vi "GPS显示界面.vi"() -> ()   [LabVIEW 2016, in "环境动力监测库.lvlib" / "NMEA.lvlib"]
uses:
  NMEA.lvlib
  NMEA_GPVTG-data.ctl
  NMEA_Mode.ctl
  NMEA_GPRMC-data.ctl
  NMEA_LatitudeDirection.ctl
  NMEA_LongitudeDirection.ctl
  NMEA_GPGGA-data.ctl
  NMEA_GPS-Quality.ctl
  <vilib>/Utility/miscctls.llb/LVPointTypeDef.ctl
  <vilib>/Utility/config.llb/NI_LVConfig.lvlib
panel:
  in  "解除告警":bool
  out "x+1":u32
  out "浮标定位点":cluster{"纬度":dbl, "经度":dbl}
  out "Port":string
  out "IP":string
  in  "手动设置定位":bool caption="定位自动获取OFF/手动设置ON"
  out "波特率":u32
  out "串口":string
  in  "移位报警设定值":dbl=1000.0
  out "GPS-Quality":T1
  out "定位状态":bool=TRUE
  in  "配置":bool
  out "Coordinates":picture
  in  "reset odometer":bool
  out "方位角 (deg)":dbl(knob) scale=0.0..360.0
  out "偏移量/米":dbl format="%#.2f"
  out "水平运动速度 (km/h)":dbl(knob) scale=0.0..180.0
  out "海拔":dbl format="%.2f"
  out "纬度":dbl
  out "经度":dbl
  out "时间":timestamp format="%<%H:%M:%S>T"
  out "日期":timestamp format="%<%Y/%m/%d>T"
  out "$GPGGA-message_OUT":T2={"TimeStamp"=timestamp(0 s since 1904-01-01), "Latitude"=0.0, "Latitude-Direction"=enum."", "Longitude"=1.0, "Longitude-Direction"=enum."", "GPS-Quality"=enum."GPS fix (SPS)", "Number of Satellites"=0, "Horizontal Dilution of Precision"=0.0, "Altitude above Mean-Sea-Level"=0.0, "Geoidal separation"=0.0, "Time since last DGPS update"=0.0, "DGPS reference station ID"=0} {"Time since last DGPS update" format="%.02f [s]"; "Geoidal separation" format="%.02f [m]"; "Altitude above Mean-Sea-Level" format="%.02f [m]"; "Horizontal Dilution of Precision" format="%.02f [HDOP]"; "Longitude" format="%0.4f [long]"; "Latitude" format="%.04f [lat]"; "TimeStamp" format="%<%.2X>T"}
  out "$GPRMC-message_OUT":T5={"TimeStamp"=timestamp(0 s since 1904-01-01), "Validity"=FALSE, "Latitude"=0.0, "Latitude-Direction"=enum."North", "Longitude"=0.0, "Longitude-Direction"=enum."East", "Speed in knots"=0.0, "True course"=0.0, "Date Stamp"=timestamp(0 s since 1904-01-01), "Magnetic Variation (East/West)"=0.0} {"Magnetic Variation (East/West)" format="%.02f [deg]"; "Date Stamp" format="%<%x>T"; "True course" format="%.02f [deg]"; "Speed in knots" format="%.02f [kts]"; "Longitude" format="%0.4f [long]"; "Latitude" format="%.04f [lat]"; "TimeStamp" format="%<%.2X>T"}
  out "$GPVTG-message_OUT":T6={"True Course over Ground"=0.0, "Magnetic Course over Ground"=0.0, "Speed over Ground in knots"=0.0, "Speed over Ground in km/h"=1.0, "Mode"=""} {"Speed over Ground in km/h" format="%.02f [km/h]"; "Speed over Ground in knots" format="%.02f [kts]"; "Magnetic Course over Ground" format="%.02f [deg]"; "True Course over Ground" format="%.02f [deg]"}
  out "Raw data GPS":string
  # "米"
  # "GPS监测"
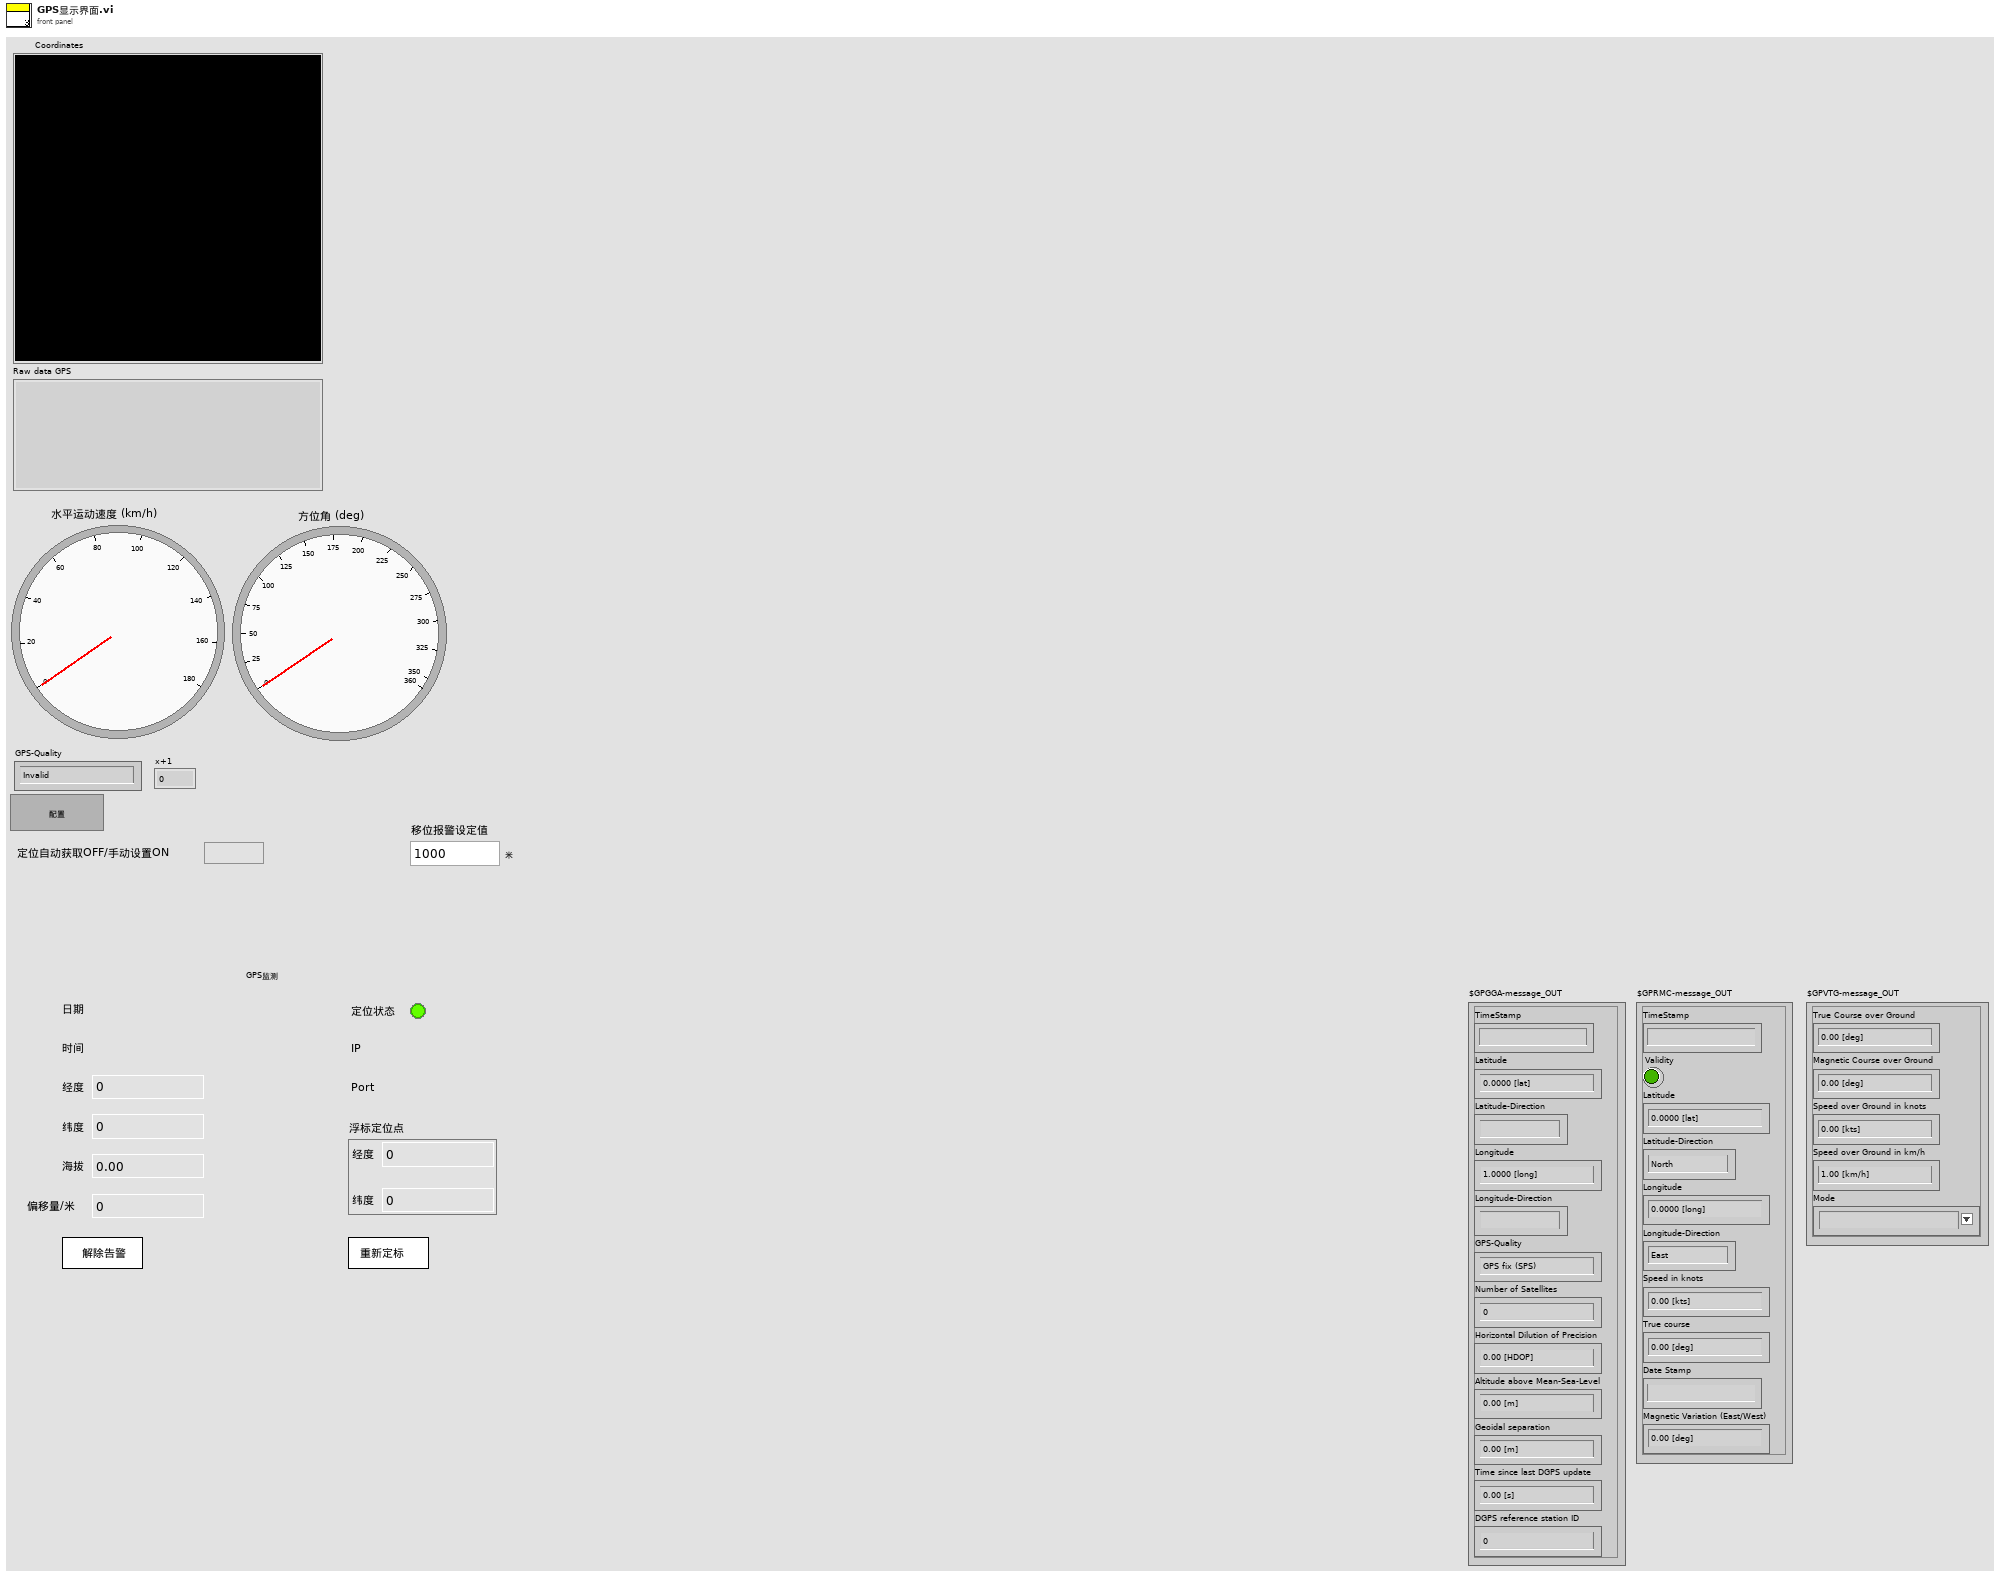
[diagram p1: front panel]
types:
  T1 = typedef "环境动力监测库.lvlib/NMEA.lvlib/NMEA_GPS-Quality.ctl" = enum16{"Invalid", "GPS fix (SPS)", "DGPS fix", "PPS fix", "Real Time Kinematic", "Float RTK", "estimated", "Manual input mode", "Simulation mode"}
  T2 = typedef "环境动力监测库.lvlib/NMEA.lvlib/NMEA_GPGGA-data.ctl" = cluster{"TimeStamp":timestamp, "Latitude":dbl, "Latitude-Direction":T3, "Longitude":dbl, "Longitude-Direction":T4, "GPS-Quality":T1, "Number of Satellites":i32, "Horizontal Dilution of Precision":dbl, "Altitude above Mean-Sea-Level":dbl, "Geoidal separation":dbl, "Time since last DGPS update":dbl, "DGPS reference station ID":i32}
  T3 = typedef "环境动力监测库.lvlib/NMEA.lvlib/NMEA_LatitudeDirection.ctl" = enum16{"", "North", "South"}
  T4 = typedef "环境动力监测库.lvlib/NMEA.lvlib/NMEA_LongitudeDirection.ctl" = enum16{"", "East", "West"}
  T5 = typedef "环境动力监测库.lvlib/NMEA.lvlib/NMEA_GPRMC-data.ctl" = cluster{"TimeStamp":timestamp, "Validity":bool, "Latitude":dbl, "Latitude-Direction":T3, "Longitude":dbl, "Longitude-Direction":T4, "Speed in knots":dbl, "True course":dbl, "Date Stamp":timestamp, "Magnetic Variation (East/West)":dbl}
  T6 = typedef "环境动力监测库.lvlib/NMEA.lvlib/NMEA_GPVTG-data.ctl" = cluster{"True Course over Ground":dbl, "Magnetic Course over Ground":dbl, "Speed over Ground in knots":dbl, "Speed over Ground in km/h":dbl, "Mode":T7}
  T7 = typedef "环境动力监测库.lvlib/NMEA.lvlib/NMEA_Mode.ctl" = string
  T8 = cluster{"监测项描述:输出":string, "连接方式":enum16{"串口", "TCP"}, "端口":string, "IP address:":string, "Port:":string, "站号":u64, "传感器型号":string, "波特率":u64, "data bits":u64, "停止位":u16, "奇偶校验":u16, "声光告警启用":bool}
  T9 = typedef "LVPointTypeDef.ctl" = cluster{"Horizontal":i16, "Vertical":i16}
  T10 = cluster{"定位状态":bool, "卫星数量":u16, "时间标识":timestamp, "纬度":dbl, "南北":string, "经度":dbl, "东西":string}
  T11 = cluster{"网络参数":cluster{"网络状态":bool, "本机IP":string[]}, "电源管理":cluster{"电源管理":bool, "氨氮电源":bool, "总磷电源":bool, "总氮电源":bool, "多参数电源":bool, "CODMn电源":bool, "CODCr电源":bool, "灯带电源":bool, "照明电源":bool}, "北斗-GPS":cluster{"GPS":cluster{"经度:":sgl, "纬度: ":sgl, "GPS监测":bool}, "北斗":cluster{"经度:":sgl, "纬度:":sgl, "北斗监测":bool}}}
  T12 = typedef "NI_LVConfig.lvlib/Config Data RefNum.ctl" = refnum<k1>
  T13 = cluster{"漏水监测输出":cluster{"漏水监测告警":bool, "告警内容":string}, "门禁监测输出":cluster{"门禁监测告警":bool, "告警内容":string}, "门禁监测输出2":cluster{"门禁监测告警":bool, "告警内容":string}, "温湿度监测输出":cluster{"温湿度监测告警":bool, "告警内容":string}, "烟雾监测输出":cluster{"烟雾监测告警":bool, "告警内容":string}, "空调监测输出":cluster{"空调监测告警":bool, "告警内容":string}, "自动重合闸输出":cluster{"自动重合闸告警":bool, "告警内容":string}, "红外入侵输出":cluster{"红外入侵告警":bool, "告警内容":string}, "振动输出":cluster{"振动告警":bool, "告警内容":string}, "UPS输出":cluster{"UPS告警":bool, "告警内容":string}, "蓄电池输出":cluster{"蓄电池告警":bool, "告警内容":string}, "蓄电池输出2":cluster{"蓄电池告警":bool, "告警内容":string}, "GPS输出":cluster{"定位告警":bool, "告警内容":string}, "北斗输出":cluster{"定位告警":bool, "告警内容":string}, "气象输出":cluster{"气象告警":bool, "告警内容":string}}
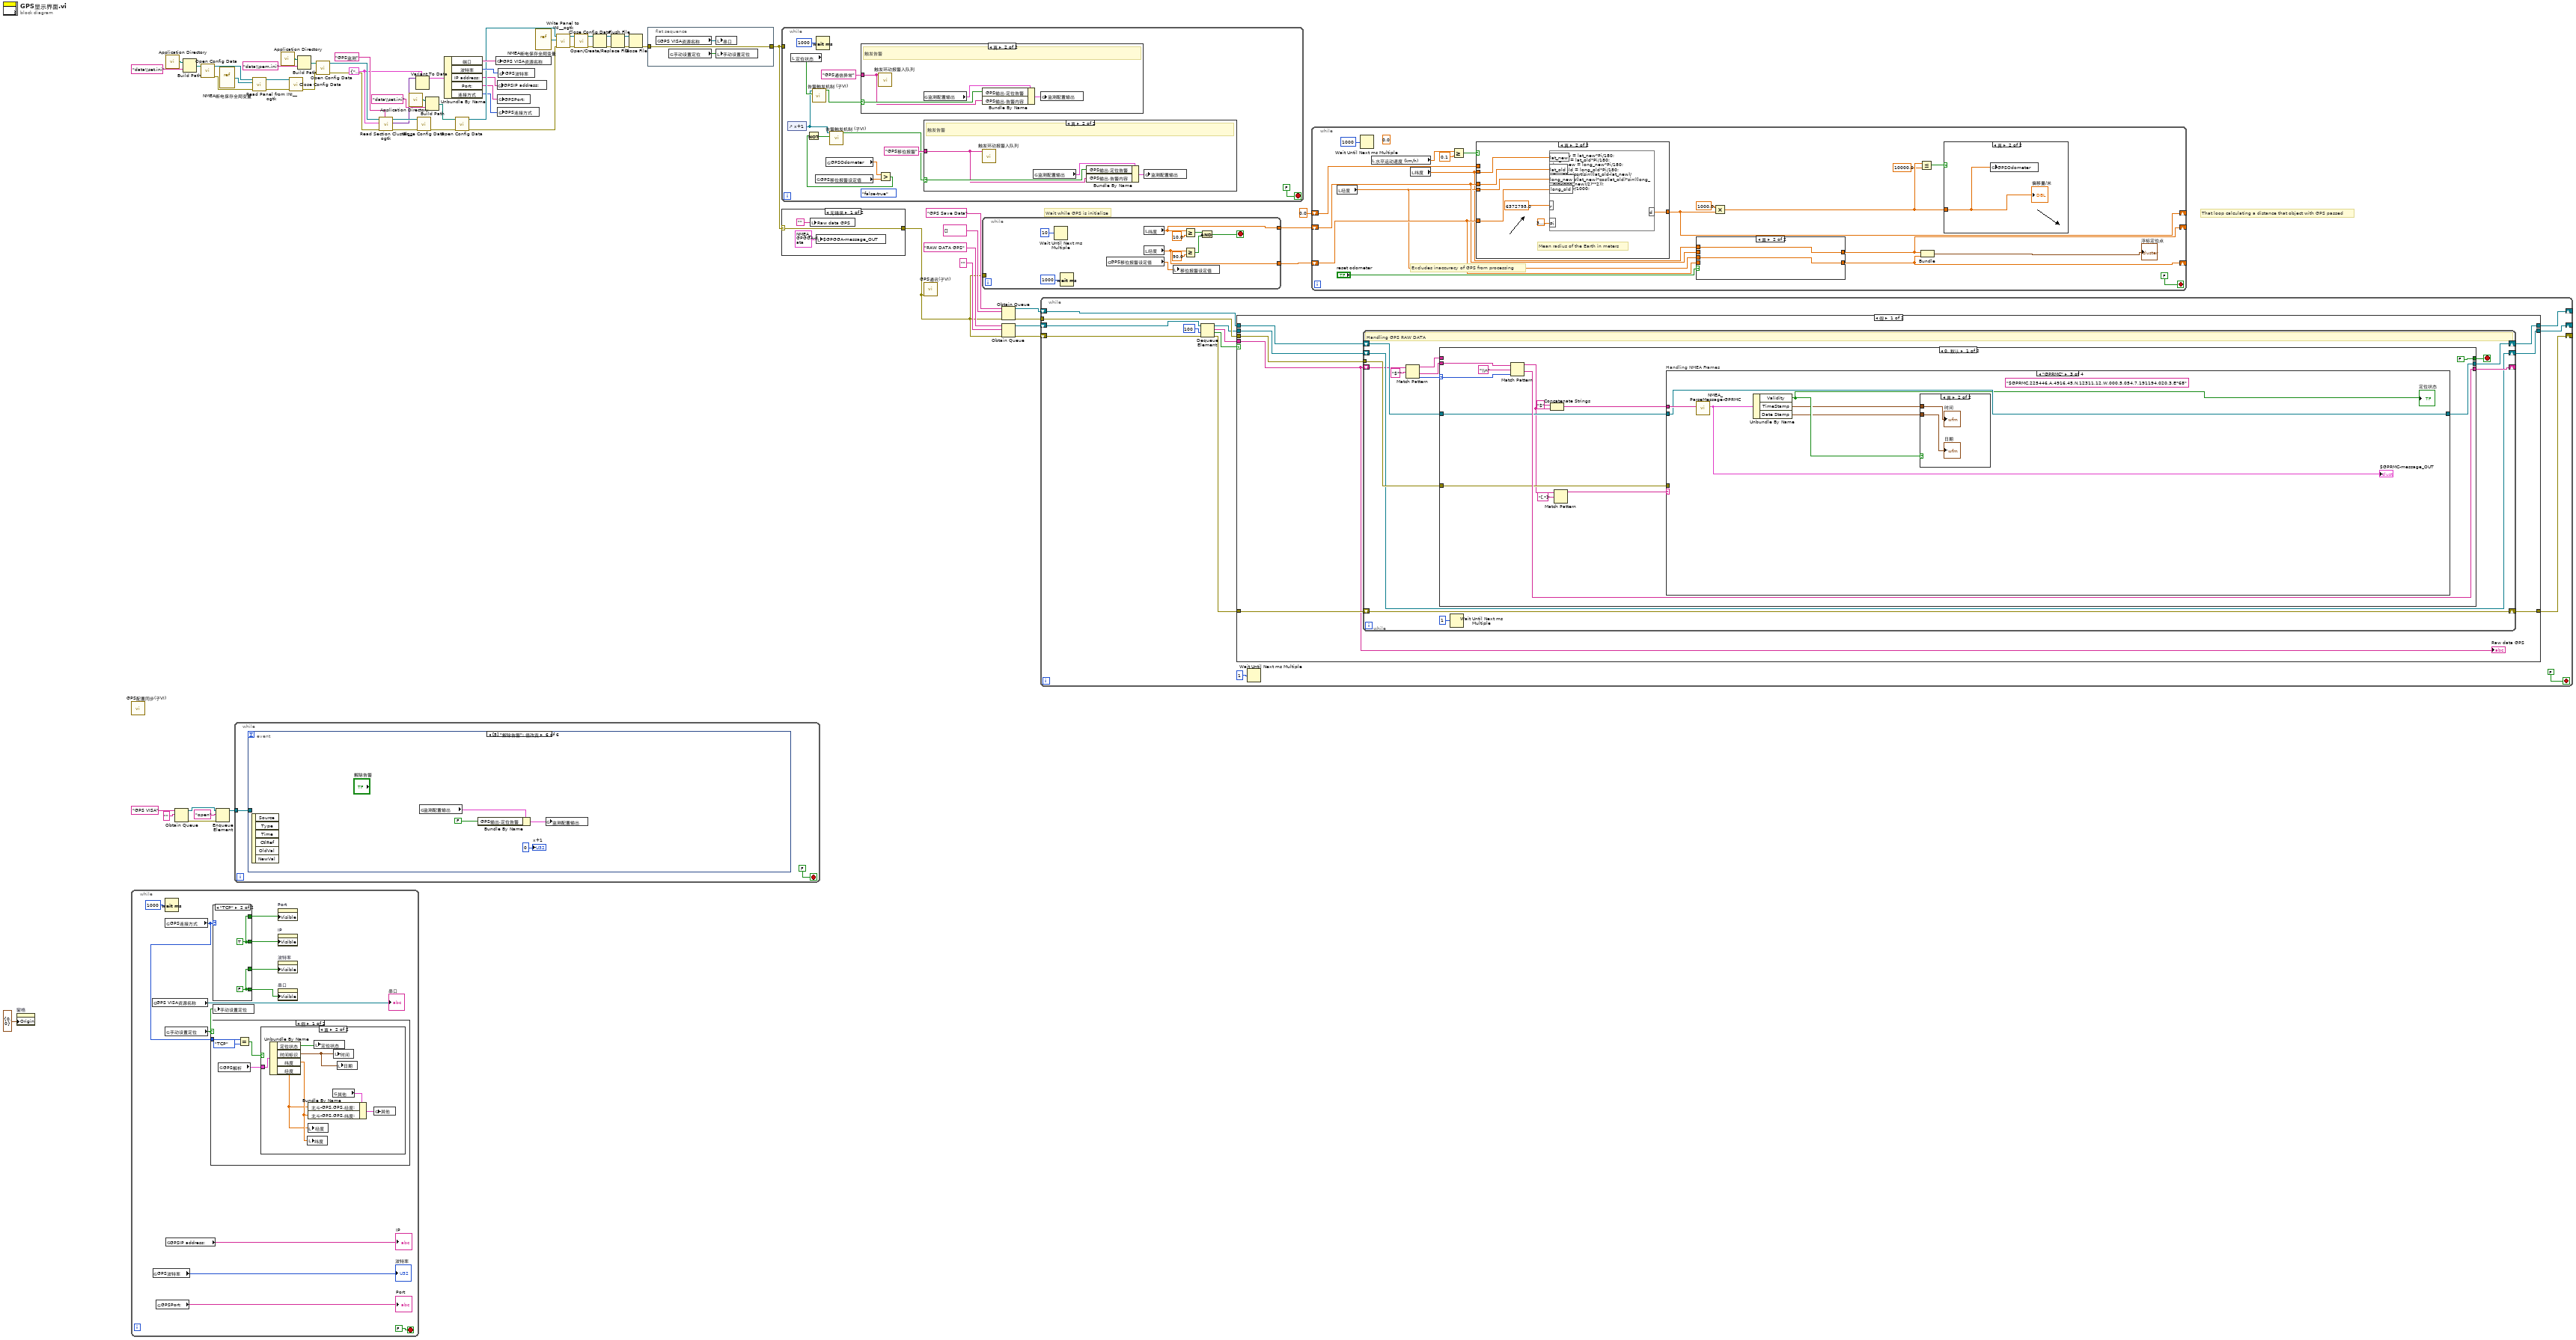
[diagram p0: block diagram]
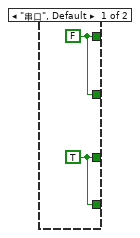
[diagram p4: hidden frame]
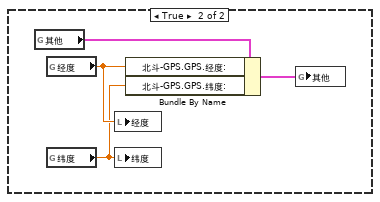
[diagram p6: hidden frame]
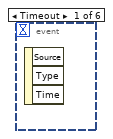
[diagram p7: hidden frame]
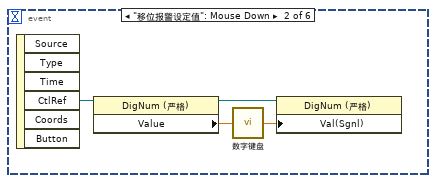
[diagram p8: hidden frame]
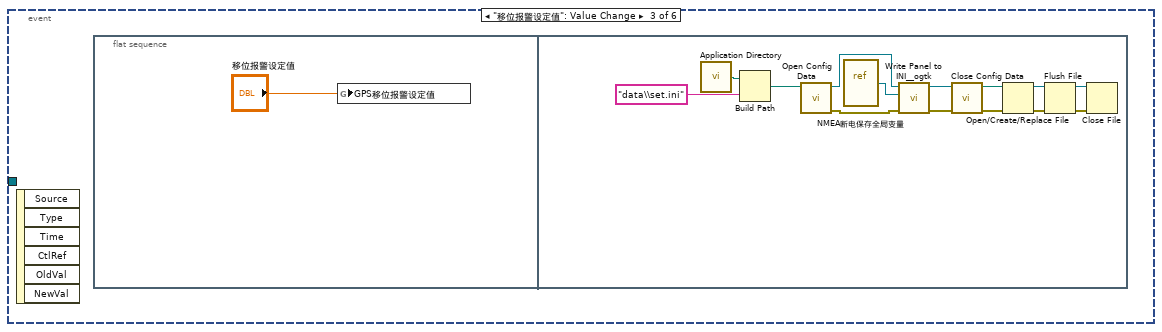
[diagram p9: hidden frame]
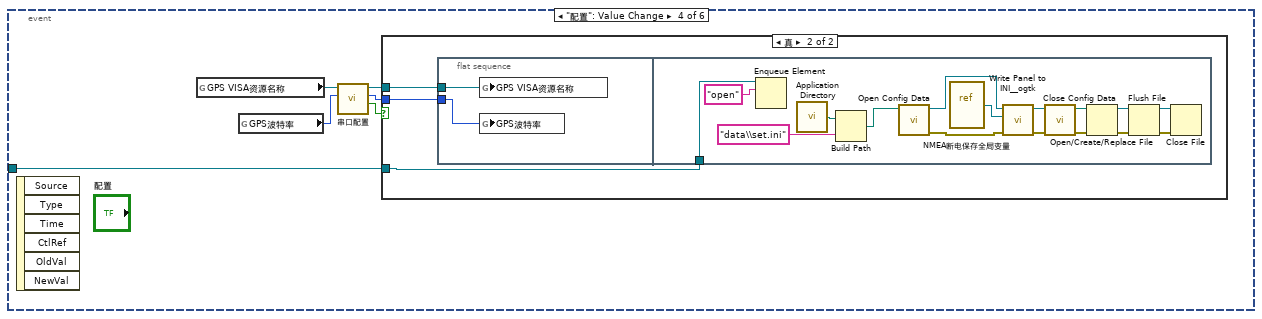
[diagram p10: hidden frame]
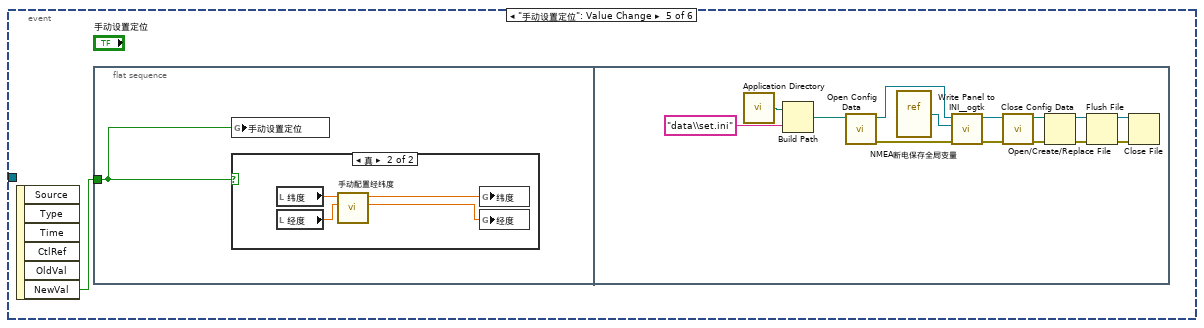
[diagram p12: hidden frame]
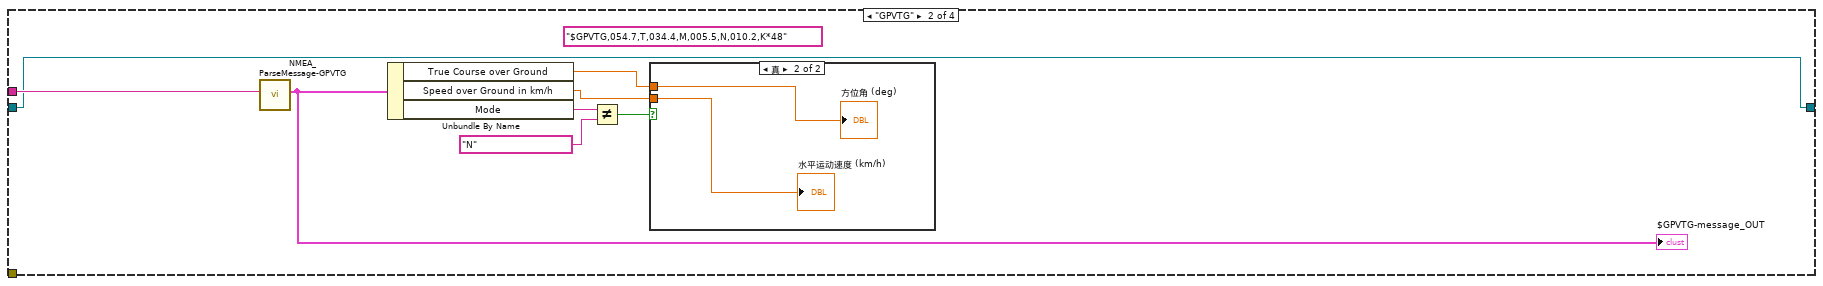
[diagram p19: hidden frame]
diagram:
  w22 = T8 {"监测项描述:输出"="", "连接方式"=enum."串口", "端口"="", "IP address:"="", "Port:"="", "站号"=19200, "传感器型号"="", "波特率"=19200, "data bits"=8, "停止位"=10, "奇偶校验"=0, "声光告警启用"=FALSE} ("输入簇")
  (unwired) 0.0 ("方位角 (deg)")
  # "That loop calculating a distance that object with GPS passed"
  # "Wait while GPS is initialize"
  n1 = property on="窗格" class="Pane"("Origin"=T9 {"Horizontal"=0, "Vertical"=0} ("原点")) -> ()  [unwired: 2 in, 2 out]
  n2 = call "GPS配置同步(子VI).vi"() -> ()  [unwired: 12 in]
  n3 = while {
    stop <- FALSE stop-if-true
    n4 = global read "NMEA断电保存全局变量.vi" "GPS VISA资源名称"() -> (→"串口":refnum<visa-resource-name>)
    n5 = global read "NMEA断电保存全局变量.vi" "GPS波特率"() -> (→"波特率":u32)
    n6 = global read "NMEA断电保存全局变量.vi" "GPSPort:"() -> (→"Port":string)
    n7 = Wait (ms)(milliseconds to wait=u32 1000 ("等待时间（毫秒）")) -> ()  [unwired: 1 out]
    n8 = global read "NMEA断电保存全局变量.vi" "GPS连接方式"() -> (w62:enum16{"串口", "TCP"})
    n9 = global read "NMEA断电保存全局变量.vi" "手动设置定位"() -> (w69:bool)
    n10 = global read "NMEA断电保存全局变量.vi" "GPSIP address:"() -> (→"IP":string)
    n11 = case shown="假" w69 {
      tunnel: w62 -> [w81 _]
      frame False {
        n12 = global read "NMEA过程全局变量.vi" "GPS解析"() -> (w78:T10)
        n13 = Equal?(x=w81, y=enum16{"串口", "TCP"}."TCP") -> (x = y?=w79:bool)
        n14 = case shown="真" w79 {
          tunnel: w78 -> [_ w88]
          frame False {
          }
          frame True {
            n15 = Unbundle By Name(w88) -> ("定位状态"=w87:bool, "时间标识"=w86:timestamp, "纬度"=w83:dbl, "经度"=w82:dbl)
            n16 = local write "纬度"(w83) -> ()
            n17 = local write "经度"(w82) -> ()
            n18 = local write "定位状态"(w87) -> ()
            n19 = global read "内部交互全局变量.vi" "其他"() -> (w85:T11)
            n20 = Bundle By Name(cluster=w85, "北斗-GPS.GPS.经度:"=w82, "北斗-GPS.GPS.纬度:"=w83) -> (w84:T11)
            n21 = local write "时间"(w86) -> ()
            n22 = local write "日期"(w86) -> ()
            n23 = global write "内部交互全局变量.vi" "其他"(w84) -> ()
          }
        }
      }
      frame True {
        n24 = global read "内部交互全局变量.vi" "其他"() -> (w92:T11)
        n25 = global read "NMEA断电保存全局变量.vi" "经度"() -> (w90:dbl)
        n26 = global read "NMEA断电保存全局变量.vi" "纬度"() -> (w89:dbl)
        n27 = local write "经度"(w90) -> ()
        n28 = local write "纬度"(w89) -> ()
        n29 = Bundle By Name(cluster=w92, "北斗-GPS.GPS.经度:"=w90, "北斗-GPS.GPS.纬度:"=w89) -> (w91:T11)
        n30 = global write "内部交互全局变量.vi" "其他"(w91) -> ()
      }
    }
    n31 = case shown="\"TCP\"" w62 {
      tunnel: [w75 w77] -> w66
      tunnel: [w75 w77] -> w65
      tunnel: [w74 w76] -> w64
      tunnel: [w74 w76] -> w63
      frame "串口", Default {
        w74 = FALSE
        w75 = TRUE
      }
      frame "TCP" {
        w76 = TRUE
        w77 = FALSE
      }
    }
    n32 = local write "手动设置定位"(w69) -> ()
    n33 = property on="Port" class="Str"("Visible"=w63) -> ()  [unwired: 2 in, 2 out]
    n34 = property on="IP" class="Str"("Visible"=w64) -> ()  [unwired: 2 in, 2 out]
    n35 = property on="波特率" class="DigNum (严格)"("Visible"=w65) -> ()  [unwired: 2 in, 2 out]
    n36 = property on="串口" class="Str"("Visible"=w66) -> ()  [unwired: 2 in, 2 out]
  }
  n37 = call <vilib>:"Application Directory.vi"() -> ("Application Directory"=w35:path)
  n38 = Obtain Queue(name (unnamed)="GPS VISA" ("名称（未命名）"), element data type="" ("名称（未命名）")) -> (queue out=w45:refnum<queue>, error out=w44:errorcluster)  [unwired: 3 in, 1 out]
  n39 = Build Path(base path=w35, name or relative path="data\\set.ini" ("名称或相对路径")) -> (appended path=w34:path)
  n40 = call <vilib>:"Open Config Data.vi"("configuration file path"=w34) -> ("error out"=w38:errorcluster, "refnum"=w37:T12)  [unwired: 8 in, 1 out]
  n41 = Enqueue Element(queue=w45, element="open" ("元素"), error in (no error)=w44) -> (queue out=w42:refnum<queue>)  [unwired: 1 in, 2 out]
  n42 = vi-ref "NMEA断电保存全局变量.vi"() -> (w33:refnum<vi>)
  n43 = while {
    tunnel: w42 -> [w94]
    stop <- FALSE stop-if-true
    n44 = event shown="[5] \"解除告警\": 值改变" {
      selector: _ -> [_ _ _ _ _ _]
      dyn-events: _ -> [_ _ _ _ _ _]
      timeout: _ -> [_ _ _ _ _ _]
      tunnel: w94 -> [_ _ _ w114 _ _]
      event Timeout {
        n45 = event-data() -> ()  [unwired: 1 in, 3 out]
      }
      event "移位报警设定值": Mouse Down {
        n46 = event-data() -> ("CtlRef"=w95:refnum<vi>)  [unwired: 1 in, 5 out]
        n47 = property class="DigNum (严格)"(reference=w95) -> (reference out=w96:refnum<vi>, "Value"=w98:dbl)  [unwired: 1 in, 1 out]
        n48 = call "数字键盘.vi"("OldNumber"=w98) -> ("NewNumber"=w97:dbl)
        n49 = property class="DigNum (严格)"(reference=w96, "Val(Sgnl)"=w97) -> ()  [unwired: 1 in, 2 out]
      }
      event "移位报警设定值": Value Change {
        n50 = event-data() -> ()  [unwired: 1 in, 6 out]
        n51 = flat-sequence {
          frame #0 {
            n52 = global write "NMEA断电保存全局变量.vi" "GPS移位报警设定值"("移位报警设定值") -> ()
          }
          frame #1 {
            n53 = call <vilib>:"Application Directory.vi"() -> ("Application Directory"=w112:path)
            n54 = Build Path(base path=w112, name or relative path="data\\set.ini" ("名称或相对路径")) -> (appended path=w113:path)
            n55 = call <vilib>:"Open Config Data.vi"("configuration file path"=w113) -> ("error out"=w109:errorcluster, "refnum"=w110:T12)  [unwired: 8 in, 1 out]
            n56 = vi-ref "NMEA断电保存全局变量.vi"() -> (w106:refnum<vi>)
            n57 = call <userlib>:"Write Panel to INI__ogtk.vi"("error in (no error)"=w109, "VI ref"=w106, "refnum"=w110) -> ("error out"=w107:errorcluster, "refnum out"=w108:T12)  [unwired: 7 in]
            n58 = call <vilib>:"Close Config Data.vi"("error in (no error)"=w107, "refnum"=w108) -> ("error out"=w105:errorcluster, "file path"=w104:path)  [unwired: 8 in]
            n59 = Open/Create/Replace File(file path (use dialog)=w104, error in=w105) -> (refnum out=w102:refnum<file>, error out=w103:errorcluster)  [unwired: 4 in, 1 out]
            n60 = Flush File(refnum=w102, error in=w103) -> (refnum out=w100:refnum<file>, error out=w101:errorcluster)
            n61 = Close File(refnum=w100, error in=w101) -> ()  [unwired: 2 out]
          }
        }
      }
      event "配置": Value Change {
        n62 = event-data() -> ()  [unwired: 1 in, 6 out]
        n63 = global read "NMEA断电保存全局变量.vi" "GPS VISA资源名称"() -> (w117:refnum<visa-resource-name>)
        n64 = global read "NMEA断电保存全局变量.vi" "GPS波特率"() -> (w115:u32)
        n65 = call "串口配置.vi"("波特率"=w115, "VISA资源名称"=w117) -> ("确认 2"=w119:bool, "波特率输出"=w116:u32, "VISA资源名称 2"=w118:refnum<visa-resource-name>)  [unwired: 7 in]
        n66 = case shown="真" w119 {
          tunnel: w118 -> [_ w122]
          tunnel: w116 -> [_ w121]
          tunnel: w114 -> [_ w120]
          frame False {
          }
          frame True {
            n67 = flat-sequence {
              tunnel: w122 -> [w124]
              tunnel: w121 -> [w123]
              tunnel: w120 -> [w126]
              frame #0 {
                n68 = global write "NMEA断电保存全局变量.vi" "GPS VISA资源名称"(w124) -> ()
                n69 = global write "NMEA断电保存全局变量.vi" "GPS波特率"(w123) -> ()
              }
              frame #1 {
                n70 = Enqueue Element(queue=w126, element="open" ("元素")) -> ()  [unwired: 2 in, 3 out]
                n71 = call <vilib>:"Application Directory.vi"() -> ("Application Directory"=w139:path)
                n72 = Build Path(base path=w139, name or relative path="data\\set.ini" ("名称或相对路径")) -> (appended path=w140:path)
                n73 = call <vilib>:"Open Config Data.vi"("configuration file path"=w140) -> ("error out"=w136:errorcluster, "refnum"=w137:T12)  [unwired: 8 in, 1 out]
                n74 = vi-ref "NMEA断电保存全局变量.vi"() -> (w133:refnum<vi>)
                n75 = call <userlib>:"Write Panel to INI__ogtk.vi"("error in (no error)"=w136, "VI ref"=w133, "refnum"=w137) -> ("error out"=w134:errorcluster, "refnum out"=w135:T12)  [unwired: 7 in]
                n76 = call <vilib>:"Close Config Data.vi"("error in (no error)"=w134, "refnum"=w135) -> ("error out"=w132:errorcluster, "file path"=w131:path)  [unwired: 8 in]
                n77 = Open/Create/Replace File(file path (use dialog)=w131, error in=w132) -> (refnum out=w129:refnum<file>, error out=w130:errorcluster)  [unwired: 4 in, 1 out]
                n78 = Flush File(refnum=w129, error in=w130) -> (refnum out=w127:refnum<file>, error out=w128:errorcluster)
                n79 = Close File(refnum=w127, error in=w128) -> ()  [unwired: 2 out]
              }
            }
          }
        }
      }
      event "手动设置定位": Value Change {
        n80 = event-data() -> ("NewVal"=w141:bool)  [unwired: 1 in, 5 out]
        n81 = flat-sequence {
          tunnel: w141 -> [w142]
          frame #0 {
            n82 = global write "NMEA断电保存全局变量.vi" "手动设置定位"(w142) -> ()
            n83 = case shown="真" w142 {
              frame False {
              }
              frame True {
                n84 = local read "纬度"() -> (w146:dbl)
                n85 = local read "经度"() -> (w145:dbl)
                n86 = call "手动配置经纬度.vi"("经度输入"=w145, "纬度输入"=w146) -> ("经度"=w143:dbl, "纬度"=w144:dbl)  [unwired: 8 in]
                n87 = global write "NMEA断电保存全局变量.vi" "纬度"(w144) -> ()
                n88 = global write "NMEA断电保存全局变量.vi" "经度"(w143) -> ()
              }
            }
          }
          frame #1 {
            n89 = call <vilib>:"Application Directory.vi"() -> ("Application Directory"=w159:path)
            n90 = Build Path(base path=w159, name or relative path="data\\set.ini" ("名称或相对路径")) -> (appended path=w160:path)
            n91 = call <vilib>:"Open Config Data.vi"("configuration file path"=w160) -> ("error out"=w156:errorcluster, "refnum"=w157:T12)  [unwired: 8 in, 1 out]
            n92 = vi-ref "NMEA断电保存全局变量.vi"() -> (w153:refnum<vi>)
            n93 = call <userlib>:"Write Panel to INI__ogtk.vi"("error in (no error)"=w156, "VI ref"=w153, "refnum"=w157) -> ("error out"=w154:errorcluster, "refnum out"=w155:T12)  [unwired: 7 in]
            n94 = call <vilib>:"Close Config Data.vi"("error in (no error)"=w154, "refnum"=w155) -> ("error out"=w152:errorcluster, "file path"=w151:path)  [unwired: 8 in]
            n95 = Open/Create/Replace File(file path (use dialog)=w151, error in=w152) -> (refnum out=w149:refnum<file>, error out=w150:errorcluster)  [unwired: 4 in, 1 out]
            n96 = Flush File(refnum=w149, error in=w150) -> (refnum out=w147:refnum<file>, error out=w148:errorcluster)
            n97 = Close File(refnum=w147, error in=w148) -> ()  [unwired: 2 out]
          }
        }
      }
      event "解除告警": Value Change {
        n98 = event-data() -> ()  [unwired: 1 in, 6 out]
        n99 = global read "断电保存全局变量.vi" "监测配置输出"() -> (w163:T13)
        n100 = Bundle By Name(cluster=w163, "GPS输出.定位告警"=FALSE) -> (w164:T13)
        n101 = global write "断电保存全局变量.vi" "监测配置输出"(w164) -> ()
        "x+1" <- u32 0 ("x+1")
      }
    }
  }
  n102 = call <userlib>:"Read Panel from INI__ogtk.vi"("error in (no error)"=w38, "VI ref"=w33, "refnum"=w37) -> ("error out"=w40:errorcluster, "refnum out"=w39:T12)  [unwired: 7 in]
  n103 = call <vilib>:"Application Directory.vi"() -> ("Application Directory"=w29:path)
  n104 = call <vilib>:"Close Config Data.vi"("error in (no error)"=w40, "refnum"=w39) -> ("error out"=w5:errorcluster)  [unwired: 8 in, 1 out]
  n105 = Build Path(base path=w29, name or relative path="data\\pem.ini" ("名称或相对路径")) -> (appended path=w30:path)
  n106 = call <vilib>:"Open Config Data.vi"("error in (no error)"=w5, "configuration file path"=w30) -> ("error out"=w31:errorcluster, "refnum"=w32:T12)  [unwired: 7 in, 1 out]
  n107 = call <userlib>:"Read Section Cluster__ogtk.vi"("section (optional)"="GPS监测", "error in (no error)"=w31, "Section Formatted Cluster Type"=w22, "refnum"=w32) -> ("error out"=w25:errorcluster, "Section Formatted Cluster"=w24:variant, "dup refnum"=w26:T12)  [unwired: 3 in, 2 out]
  n108 = call <vilib>:"Application Directory.vi"() -> ("Application Directory"=w18:path)
  n109 = Variant To Data(type=w22, Variant=w24) -> (data=w23:T8)  [unwired: 1 in, 1 out]
  n110 = call <vilib>:"Close Config Data.vi"("error in (no error)"=w25, "refnum"=w26) -> ("error out"=w4:errorcluster)  [unwired: 8 in, 1 out]
  n111 = Build Path(base path=w18, name or relative path="data\\set.ini" ("名称或相对路径")) -> (appended path=w19:path)
  n112 = Unbundle By Name(w23) -> ("端口"=w21:string, "波特率"=w20:u64, "IP address:"=w3:string, "Port:"=w2:string, "连接方式"=w1:enum16{"串口", "TCP"})
  n113 = call <vilib>:"Open Config Data.vi"("error in (no error)"=w4, "configuration file path"=w19) -> ("error out"=w15:errorcluster, "refnum"=w16:T12)  [unwired: 7 in, 1 out]
  n114 = global write "NMEA断电保存全局变量.vi" "GPS VISA资源名称"(w21) -> ()
  n115 = global write "NMEA断电保存全局变量.vi" "GPSIP address:"(w3) -> ()
  n116 = global write "NMEA断电保存全局变量.vi" "GPSPort:"(w2) -> ()
  n117 = global write "NMEA断电保存全局变量.vi" "GPS连接方式"(w1) -> ()
  n118 = global write "NMEA断电保存全局变量.vi" "GPS波特率"(w20) -> ()
  n119 = vi-ref "NMEA断电保存全局变量.vi"() -> (w12:refnum<vi>)
  n120 = call <userlib>:"Write Panel to INI__ogtk.vi"("error in (no error)"=w15, "VI ref"=w12, "refnum"=w16) -> ("error out"=w13:errorcluster, "refnum out"=w14:T12)  [unwired: 7 in]
  n121 = call <vilib>:"Close Config Data.vi"("error in (no error)"=w13, "refnum"=w14) -> ("error out"=w11:errorcluster, "file path"=w10:path)  [unwired: 8 in]
  n122 = Open/Create/Replace File(file path (use dialog)=w10, error in=w11) -> (refnum out=w8:refnum<file>, error out=w9:errorcluster)  [unwired: 4 in, 1 out]
  n123 = Flush File(refnum=w8, error in=w9) -> (refnum out=w6:refnum<file>, error out=w7:errorcluster)
  n124 = Close File(refnum=w6, error in=w7) -> (error out=w49:errorcluster)  [unwired: 1 out]
  n125 = flat-sequence {
    tunnel: w49 -> [w166]
    tunnel: [w166] -> w48
    frame #0 {
      n126 = global read "NMEA断电保存全局变量.vi" "GPS VISA资源名称"() -> (w167:refnum<visa-resource-name>)
      n127 = global read "NMEA断电保存全局变量.vi" "手动设置定位"() -> (w165:bool)
      n128 = local write "串口"(w167) -> ()
      n129 = local write "手动设置定位"(w165) -> ()
    }
  }
  n130 = while {
    tunnel: w48 -> [_]
    stop <- FALSE stop-if-true
    (unwired) enum16{"either", "false-true", "true-false"}."false-true" ("direction")
    n131 = control-ref of="x+1"() -> (w169:refnum<vi>)
    n132 = local read "定位状态"() -> (w170:bool)
    n133 = call "告警触发机制 (子VI).vi"("状态输出"=w170, "Digital输入"=w169) -> ("触发告警"=w168:bool)  [unwired: 8 in, 1 out]
    n134 = global read "NMEA断电保存全局变量.vi" "GPS移位报警设定值"() -> (w177:dbl)
    n135 = Wait (ms)(milliseconds to wait=u32 1000 ("等待时间（毫秒）")) -> ()  [unwired: 1 out]
    n136 = global read "NMEA过程全局变量.vi" "GPSOdometer"() -> (w178:dbl)
    n137 = case shown="真" w168 {
      selector: w168 -> [_ w181]
      tunnel: "GPS通信异常" ("设备") -> [_ w180]
      frame False {
      }
      frame True {
        # "触发告警"
        n138 = call "触发环动报警入队列.vi"("报警内容"=w180) -> ()  [unwired: 11 in]
        n139 = global read "断电保存全局变量.vi" "监测配置输出"() -> (w182:T13)
        n140 = Bundle By Name(cluster=w182, "GPS输出.定位告警"=w181, "GPS输出.告警内容"=w180) -> (w183:T13)
        n141 = global write "断电保存全局变量.vi" "监测配置输出"(w183) -> ()
      }
    }
    n142 = Greater?(x=w178, y=w177) -> (0:w172:bool)
    n143 = Not(x=w172) -> (.not. x?=w173:bool)
    n144 = call "告警触发机制 (子VI).vi"("状态输出"=w173, "Digital输入"=w169) -> ("触发告警"=w171:bool)  [unwired: 8 in, 1 out]
    n145 = case shown="真" w171 {
      selector: w171 -> [_ w185]
      tunnel: "GPS移位报警" ("设备") -> [_ w184]
      frame False {
      }
      frame True {
        # "触发告警"
        n146 = call "触发环动报警入队列.vi"("报警内容"=w184) -> ()  [unwired: 11 in]
        n147 = global read "断电保存全局变量.vi" "监测配置输出"() -> (w186:T13)
        n148 = Bundle By Name(cluster=w186, "GPS输出.定位告警"=w185, "GPS输出.告警内容"=w184) -> (w187:T13)
        n149 = global write "断电保存全局变量.vi" "监测配置输出"(w187) -> ()
      }
    }
  }
  n150 = case shown="无错误" w48 {
    selector: w48 -> [w189 w191]
    tunnel: [w189 w191] -> w41
    frame No Error {
      n151 = local write "Raw data GPS"("") -> ()
      n152 = local write "$GPGGA-message_OUT"(T2 {"TimeStamp"=timestamp(0 s since 1904-01-01), "Latitude"=0.0, "Latitude-Direction"=enum."North", "Longitude"=0.0, "Longitude-Direction"=enum."East", "GPS-Quality"=enum."Invalid", "Number of Satellites"=0, "Horizontal Dilution of Precision"=0.0, "Altitude above Mean-Sea-Level"=0.0, "Geoidal separation"=0.0, "Time since last DGPS update"=0.0, "DGPS reference station ID"=0} ("GPGGA-data")) -> ()
    }
    frame Error {
    }
  }
  n153 = call "GPS通讯(子VI).vi"("error in (no error)"=w41) -> ()  [unwired: 11 in]
  n154 = while {
    tunnel: [w196] -> w51
    tunnel: [w198] -> w52
    tunnel: w41 -> [_]
    stop <- w192 stop-if-true
    n155 = Wait Until Next ms Multiple(millisecond multiple=u32 10) -> ()  [unwired: 1 out]
    n156 = Wait (ms)(milliseconds to wait=u32 1000 ("等待时间（毫秒）")) -> ()  [unwired: 1 out]
    n157 = global read "NMEA断电保存全局变量.vi" "GPS移位报警设定值"() -> (w200:dbl)
    n158 = local read "纬度"() -> (w198:dbl)
    n159 = local read "经度"() -> (w196:dbl)
    n160 = local write "移位报警设定值"(w200) -> ()
    n161 = Greater Or Equal?(x=w198, y=10.0) -> (x >= y?=w193:bool)
    n162 = Greater Or Equal?(x=w196, y=90.0) -> (x >= y?=w194:bool)
    n163 = And(x=w193, y=w194) -> (x .and. y?=w192:bool)
  }
  n164 = Obtain Queue(name (unnamed)="GPS Save Data" ("名称（未命名）"), element data type=string[] [], error in (no error)=w41) -> (queue out=w60:refnum<queue>, error out=w59:errorcluster)  [unwired: 2 in, 1 out]
  n165 = Obtain Queue(name (unnamed)="RAW DATA GPS" ("nom (aucun)"), element data type="" ("expression régulière"), error in (no error)=w41) -> (queue out=w57:refnum<queue>, error out=w61:errorcluster)  [unwired: 2 in, 1 out]
  n166 = while {
    tunnel: w59 -> [w211]
    shift-right: [w209] -> _
    shift-left: w57 -> [w210]
    shift-right: [w205] -> _
    shift-left: w60 -> [w212]
    shift-right: [w204] -> _
    shift-left: w61 -> [w215]
    stop <- FALSE stop-if-true
    n167 = Dequeue Element(queue=w210, timeout in ms (-1)=100 ("timeout en ms (-1)"), error in (no error)=w215) -> (queue out=w208:refnum<queue>, element=w214:string, timed out?=w206:bool, error out=w203:errorcluster)
    n168 = case shown="假" w206 {
      tunnel: w214 -> [w216 _]
      tunnel: w212 -> [w223 w318]
      tunnel: w211 -> [w222 _]
      tunnel: [w221 w319] -> w209
      tunnel: w208 -> [w220 w319]
      tunnel: [w219 w318] -> w205
      tunnel: [w218 w317] -> w204
      tunnel: w203 -> [w217 w317]
      frame False {
        n169 = while {
          shift-right: [w234] -> _
          shift-left: w216 -> [w225]
          tunnel: w222 -> [w230]
          shift-right: [w229] -> w221
          shift-left: w220 -> [w229]
          shift-right: [w227] -> w219
          shift-left: w223 -> [w231]
          shift-right: [w226] -> w218
          shift-left: w217 -> [w226]
          stop <- w228 stop-if-true
          # "Handling GPS RAW DATA"
          n170 = Match Pattern(string=w225, regular expression="$*" ("expression régulière")) -> (before substring=w224:string, after substring=w233:string, offset past match=w235:i32)  [unwired: 1 in, 1 out]
          n171 = case shown="0, 默认" w235 {
            selector: w235 -> [w248 _]
            tunnel: [w247 w314] -> w234
            tunnel: w233 -> [w249 _]
            tunnel: [FALSE TRUE] -> w228
            tunnel: w231 -> [w243 w315]
            tunnel: w230 -> [w242 _]
            tunnel: [w240 w315] -> w227
            tunnel: w224 -> [_ w314]
            frame 0, Default {
              n172 = Match Pattern(string=w249, regular expression="\\n" ("expression régulière"), offset (0)=w248) -> (before substring=w239:string, after substring=w247:string)  [unwired: 2 out]
              n173 = Concatenate Strings("$" ("expression régulière"), w239) -> (w245:string)
              n174 = Match Pattern(string=w239, regular expression="[,*]" ("正则表达式")) -> (before substring=w237:string)  [unwired: 1 in, 3 out]
              n175 = case "Handling NMEA Frames" shown="\"GPRMC\"" w237 {
                tunnel: w245 -> [_ w258 w266 w287]
                tunnel: w243 -> [w250 w257 w265 w284]
                tunnel: w242 -> [_ _ _ w283]
                tunnel: [w250 w257 w265 w282] -> w240
                frame " ", Default {
                }
                frame "GPVTG" {
                  (unwired) "$GPVTG,054.7,T,034.4,M,005.5,N,010.2,K*48" ("$GPVTG-message_IN")
                  n176 = call "NMEA_ParseMessage-GPVTG.vi"("$GPVTG-message_IN"=w258) -> ("$GPVTG-message_OUT"=w256:T6)  [unwired: 9 in, 1 out]
                  "$GPVTG-message_OUT" <- w256
                  n177 = Unbundle By Name(w256) -> ("True Course over Ground"=w252:dbl, "Speed over Ground in km/h"=w251:dbl, "Mode"=w255:T7)
                  n178 = Not Equal?(x=w255, y=T7 "N" ("Mode")) -> (x != y?=w253:bool)
                  n179 = case shown="真" w253 {
                    tunnel: w252 -> [_ w259]
                    tunnel: w251 -> [_ w260]
                    frame False {
                    }
                    frame True {
                      "水平运动速度 (km/h)" <- w260
                      "方位角 (deg)" <- w259
                    }
                  }
                }
                frame "GPRMC" {
                  (unwired) "$GPRMC,225446,A,4916.45,N,12311.12,W,000.5,054.7,191194,020.3,E*68" ("$GPRMC-message_IN")
                  n180 = call "NMEA_ParseMessage-GPRMC.vi"("$GPRMC-message_IN"=w266) -> ("$GPRMC-message_OUT"=w264:T5)  [unwired: 9 in, 1 out]
                  "$GPRMC-message_OUT" <- w264
                  n181 = Unbundle By Name(w264) -> ("Validity"=w263:bool, "TimeStamp"=w262:timestamp, "Date Stamp"=w261:timestamp)
                  "定位状态" <- w263
                  n182 = case shown="真" w263 {
                    tunnel: w262 -> [_ w267]
                    tunnel: w261 -> [_ w268]
                    frame False {
                    }
                    frame True {
                      "时间" <- w267
                      "日期" <- w268
                    }
                  }
                }
                frame "GPGGA" {
                  (unwired) "$GPGGA,123519,4807.038,N,01131.000,E,1,08,0.9,545.4,M,46.9,M,,*47" ("data out")
                  n183 = call "NMEA_ParseMessage-GPGGA.vi"("$GPGGA-message_IN"=w287) -> ("$GPGGA-message_OUT"=w274:T2)  [unwired: 9 in, 1 out]
                  "$GPGGA-message_OUT" <- w274
                  n184 = Unbundle By Name(w274) -> ("Horizontal Dilution of Precision"=w275:dbl, "Altitude above Mean-Sea-Level"=w276:dbl, "Latitude-Direction"=w285:T3, "Latitude"=w271:dbl, "Longitude"=w273:dbl, "Longitude-Direction"=w286:T4, "GPS-Quality"=w277:T1)
                  "GPS-Quality" <- w277
                  n185 = global write "NMEA过程全局变量.vi" "GPS$GNGGA-message_OUT"(w274) -> ()
                  n186 = Greater Or Equal?(x=w271, y=1000.0) -> (x >= y?=w269:bool)
                  n187 = Greater Or Equal?(x=w273, y=9000.0) -> (x >= y?=w280:bool)
                  n188 = Equal?(x=w277, y=NMEA_GPS-Quality."GPS fix (SPS)" ("GPS-Quality")) -> (x = y?=w278:bool)
                  n189 = Compound Arithmetic op=AND(w269, w280, w278) -> (w281:bool)
                  n190 = case shown="真" w281 {
                    tunnel: w286 -> [_ w307]
                    tunnel: w271 -> [_ w301]
                    tunnel: w285 -> [_ w300]
                    tunnel: w274 -> [_ w306]
                    tunnel: w284 -> [w288 w305]
                    tunnel: w283 -> [_ w304]
                    tunnel: [w288 w303] -> w282
                    tunnel: w273 -> [_ w302]
                    tunnel: w276 -> [_ w299]
                    tunnel: w275 -> [_ _]
                    frame False {
                    }
                    frame True {
                      n191 = disable-structure shown="禁用" {
                        disable-tunnel: w306 -> [w313 _]
                        disable-tunnel: w305 -> [w312 _]
                        disable-tunnel: w304 -> [w311 _]
                        disable-tunnel: [w309 _] -> w303
                        frame Disabled {
                          n192 = call "NMEA_GPGGA_ToStringArray.vi"("$GPGGA-message_IN"=w313) -> ("$GPGGA-message_OUT"=w310:string[])  [unwired: 9 in, 1 out]
                          n193 = Enqueue Element(queue=w312, element=w310, timeout in ms (-1)=20 ("timeout en ms (-1)"), error in (no error)=w311) -> (queue out=w309:refnum<queue>)  [unwired: 2 out]
                        }
                        frame Enabled {
                        }
                      }
                      n194 = call "NMEA_Coord-ToDecimalDegrees.vi"("Longitude-Direction"=w307, "Latitude-Direction"=w300, "Longitude"=w302, "Latitude"=w301) -> ("Longitude"=w289:dbl, "Latitude"=w290:dbl)  [unwired: 6 in]
                      "经度" <- w289
                      "纬度" <- w290
                      n195 = global read "内部交互全局变量.vi" "其他"() -> (w292:T11)
                      n196 = feedback #1() -> (w295:cluster{"Longitude":dbl, "Latitude":dbl}[])  [unwired: 1 in]
                      n197 = Bundle By Name(cluster=w292, "北斗-GPS.GPS.经度:"=w289, "北斗-GPS.GPS.纬度:"=w290) -> (w291:T11)
                      n198 = Bundle("Longitude"=w289, "Latitude"=w290) -> (w297:cluster{"Longitude":dbl, "Latitude":dbl})  [unwired: 1 in]
                      n199 = Array Subset(array=w295, length=86400 ("长度")) -> (w296:cluster{"Longitude":dbl, "Latitude":dbl}[])  [unwired: 1 in]
                      n200 = Build Array (concatenate)(w297, w295) -> (w298:cluster{"Longitude":dbl, "Latitude":dbl}[])
                      n201 = feedback-in #1(w298) -> ()
                      n202 = global write "内部交互全局变量.vi" "其他"(w291) -> ()
                      n203 = call <vilib>:"Plot XY.vi"("data"=w296, "dimensions (w,h)"=cluster{"width":i16, "height":i16} {"width"=395, "height"=395}) -> ()  [unwired: 13 in, 1 out]
                      "海拔" <- w299
                    }
                  }
                }
              }
            }
            frame -1 {
            }
          }
          n204 = Wait Until Next ms Multiple(millisecond multiple=u32 1 ("n millisecondes")) -> ()  [unwired: 1 out]
        }
        "Raw data GPS" <- w216
      }
      frame True {
      }
    }
    n205 = Wait Until Next ms Multiple(millisecond multiple=u32 1 ("n millisecondes")) -> ()  [unwired: 1 out]
  }
  n206 = while {
    shift-right: [w336] -> _
    shift-left: 0.0 -> [w333]
    shift-right: [w328] -> _
    shift-left: w51 -> [w331]
    shift-right: [w329] -> _
    shift-left: w52 -> [w330]
    stop <- FALSE stop-if-true
    # "Excludes inaccuracy of GPS from processing"
    n207 = local read "经度"() -> (w326:dbl)
    n208 = Wait Until Next ms Multiple(millisecond multiple=u32 1000 ("Refresh period (ms)")) -> ()  [unwired: 1 out]
    n209 = local read "水平运动速度 (km/h)"() -> (w327:dbl)
    n210 = local read "纬度"() -> (w325:dbl)
    n211 = Greater Or Equal?(x=w327, y=0.1) -> (x >= y?=w338:bool)
    n212 = case shown="真" w338 {
      tunnel: w331 -> [_ w349]
      tunnel: w330 -> [_ w347]
      tunnel: w325 -> [_ w346]
      tunnel: w326 -> [_ w348]
      tunnel: w333 -> [w344 _]
      tunnel: [w344 w345] -> w336
      frame False {
      }
      frame True {
        # "Mean radius of the Earth in meters"
        n213 = formula code="lat_new = lat_new*Pi/180;\nlat_old = lat_old*Pi/180;\nlong_new = long_new*Pi/180;\nlong_old = long_old*Pi/180;\nd = asin(sqrt(sin((lat_old-lat_new)/2)**2+cos(lat_new)*cos(lat_old)*sin((long_old-long_new)/2)**2));\nd = 2*d*r/1000;"("Pi"=3.141592653589793, "r"=6372795.0, "long_old"=w349, "long_new"=w348, "lat_old"=w347, "lat_new"=w346) -> ("d"=w345:dbl)
      }
    }
    n214 = case shown="真" "reset odometer" {
      tunnel: w331 -> [w341 _]
      tunnel: w330 -> [w340 _]
      tunnel: w325 -> [_ w342]
      tunnel: w326 -> [_ w343]
      tunnel: [w341 w343] -> w328
      tunnel: [w340 w342] -> w329
      frame False {
      }
      frame True {
      }
    }
    n215 = Multiply(x=1000.0, y=w336) -> (x*y=w324:dbl)
    n216 = Less Or Equal?(x=w324, y=10000.0) -> (x <= y?=w322:bool)
    n217 = Bundle("纬度"=w329, "经度"=w328) -> (→"浮标定位点":cluster{"纬度":dbl, "经度":dbl})  [unwired: 1 in]
    n218 = case shown="真" w322 {
      tunnel: w324 -> [_ w339]
      frame False {
      }
      frame True {
        n219 = global write "NMEA过程全局变量.vi" "GPSOdometer"(w339) -> ()
        "偏移量/米" <- w339
      }
    }
  }
